vi "GraphXYtoFrontImagePixels.vi"(8 "error in (no error)":errorcluster, 9 "Graph Y":dbl, 10 "Graph X":dbl, 11 "IntensityGraph in":refnum<vi>) -> (0 "error out":errorcluster, 1 "Pixel Y":dbl, 2 "Pixel X":dbl, 3 "IntensityGraph out":refnum<vi>)   [LabVIEW 2023]
doc: "Translates XY graph positions into Graph's front image pixel position."
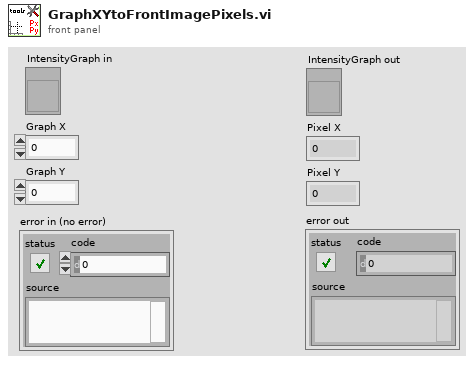
[diagram p1: front panel]
types:
  T1 = typedef "LVBoundsTypeDef.ctl" = cluster{"Width":u32, "Height":u32}
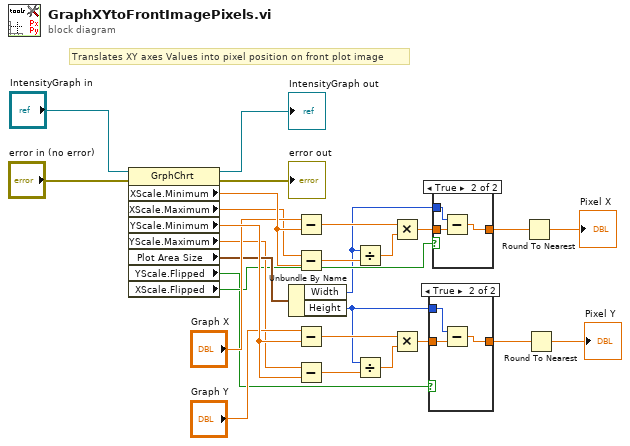
[diagram p0: block diagram]
diagram:
  # "Translates XY axes Values into pixel position on front plot image"
  n1 = property class="GrphChrt"(reference="IntensityGraph in", error in="error in (no error)") -> (reference out=→"IntensityGraph out":refnum<vi>, error out=→"error out":errorcluster, "XScale.Minimum"=w19:dbl, "XScale.Maximum"=w15:dbl, "YScale.Minimum"=w25:dbl, "YScale.Maximum"=w16:dbl, "Plot Area Size"=w17:T1, "YScale.Flipped"=w8:bool, "XScale.Flipped"=w11:bool)
  n2 = Unbundle By Name(w17) -> ("Width"=w10:u32, "Height"=w7:u32)
  n3 = Subtract(x="Graph X", y=w19) -> (x-y=w20:dbl)
  n4 = Subtract(x=w15, y=w19) -> (x-y=w21:dbl)
  n5 = Subtract(x="Graph Y", y=w25) -> (x-y=w26:dbl)
  n6 = Subtract(x=w16, y=w25) -> (x-y=w23:dbl)
  n7 = Divide(x=w10, y=w21) -> (x/y=w22:dbl)
  n8 = Divide(x=w7, y=w23) -> (x/y=w27:dbl)
  n9 = Multiply(x=w20, y=w22) -> (x*y=w12:dbl)
  n10 = Multiply(x=w26, y=w27) -> (x*y=w9:dbl)
  n11 = case shown="True" w8 {
    tunnel: w9 -> [w28 w29]
    tunnel: [w28 w31] -> w2
    tunnel: w7 -> [_ w30]
    frame False {
    }
    frame True {
      n12 = Subtract(x=w30, y=w29) -> (x-y=w31:dbl)
    }
  }
  n13 = case shown="True" w11 {
    tunnel: w12 -> [w32 w33]
    tunnel: [w32 w35] -> w4
    tunnel: w10 -> [_ w34]
    frame False {
    }
    frame True {
      n14 = Subtract(x=w34, y=w33) -> (x-y=w35:dbl)
    }
  }
  n15 = Round To Nearest(number=w4) -> (nearest integer value=→"Pixel X":dbl)
  n16 = Round To Nearest(number=w2) -> (nearest integer value=→"Pixel Y":dbl)
